vi "addCoolingBars.vi"() -> ()   [LabVIEW 2015]
uses:
  GlobalPath.vi
  GlobalData.vi
  GlobalVi.vi
panel:
  in  "Done?":bool
  in  "ptfe 2":bool caption="Position the 2 cooling bars"
  in  "Save the IDs in the database?":bool
  in  "Fill database with all cooling bar IDs?\nFill database with all 10 frame IDs?\nTo do so go to the database, select the Frame tab, choose the correct frame ID and press \"check_db\"\nThen click on \"Add/Update Entry\"":bool
  in  "COOLING BAR 2":string
  in  "COOLING BAR 1":string
  # "Add cooling bars"
  # "Associate the cooling bars to the panel in the database"
  # "Scan the ID of each of the cooling bars and associate them with the panel"
  # "Cooling bar ID recording"
  # "Fill each box with the correct IDs and press SAVE"
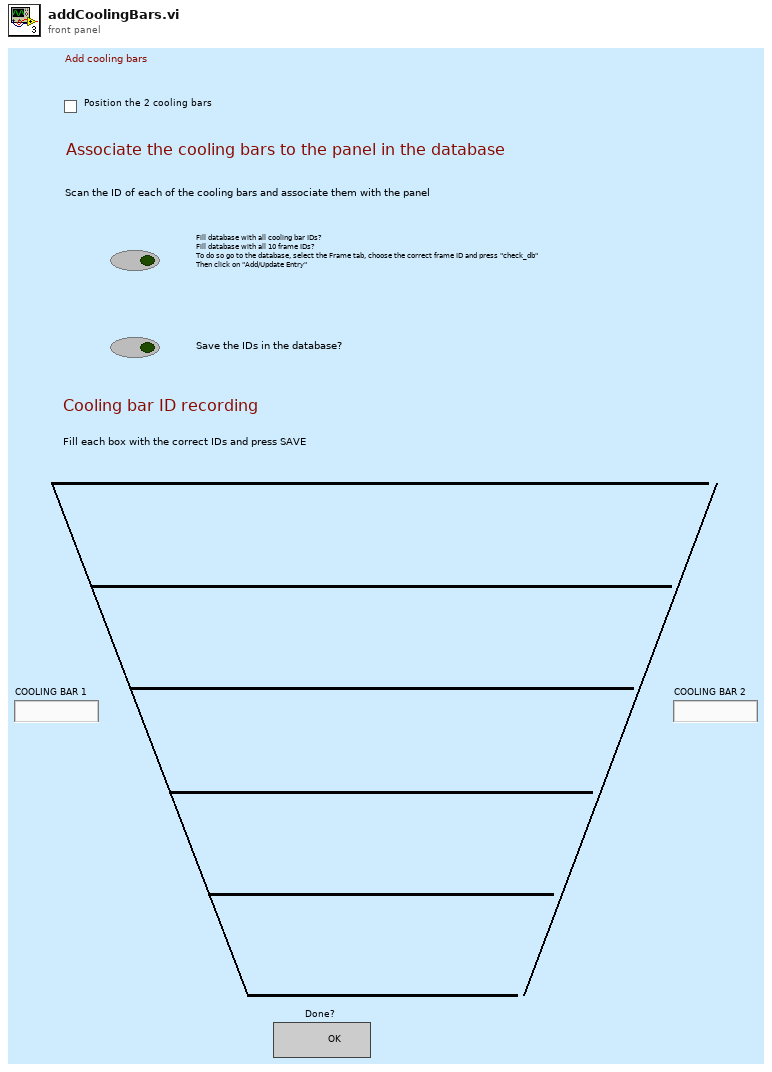
[diagram p1: front panel]
types:
  T1 = enum16{"open", "replace", "create", "open or create", "replace or create", "replace or create with confirmation"}
  T2 = enum32{"Bad", "Idle", "Run top level", "Running"}
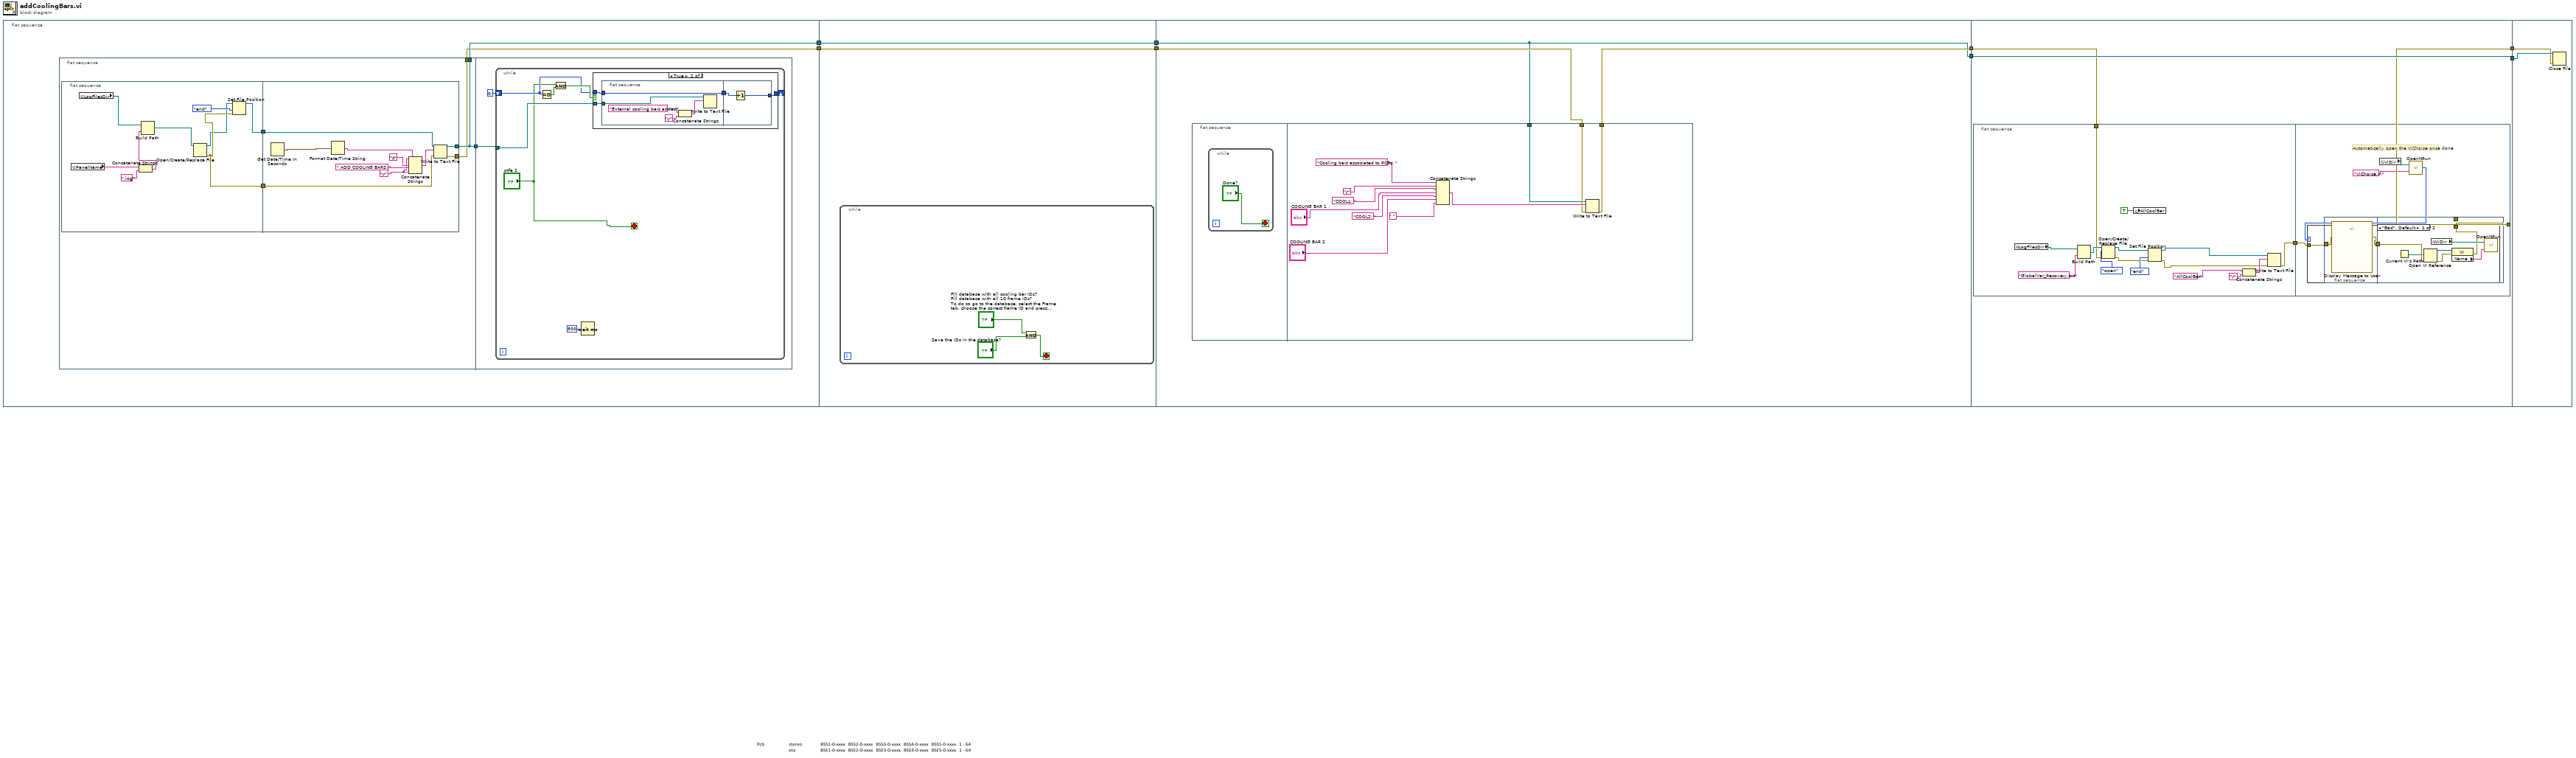
[diagram p0: block diagram]
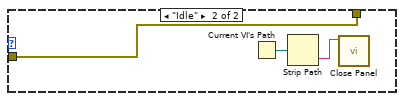
[diagram p3: hidden frame]
diagram:
  n1 = flat-sequence {
    tunnel: [w10] -> w8
    tunnel: [w9] -> w7
    tunnel: w8 -> [w57]
    tunnel: [w57] -> w2
    tunnel: w7 -> [w56]
    tunnel: [w56] -> w1
    tunnel: w2 -> [w61]
    tunnel: [w62] -> w5
    tunnel: w1 -> [w63]
    tunnel: [w61] -> w4
    tunnel: [w78] -> w6
    tunnel: w5 -> [w77]
    tunnel: w4 -> [w79]
    tunnel: [w79] -> w3
    tunnel: w6 -> [w115]
    tunnel: w3 -> [w116]
    frame #0 {
      n2 = flat-sequence {
        tunnel: [w14] -> w11
        tunnel: [w14] -> w10
        tunnel: [w13] -> w9
        tunnel: w11 -> [w36]
        frame #0 {
          n3 = flat-sequence {
            tunnel: [w17] -> w15
            tunnel: [w19] -> w12
            tunnel: w15 -> [w30]
            tunnel: [w29] -> w14
            tunnel: [w28] -> w13
            tunnel: w12 -> [w27]
            frame #0 {
              n4 = global read "GlobalData.vi" "PanelName"() -> (w23:string)
              n5 = global read "GlobalPath.vi" "LogFilesDir"() -> (w16:path)
              n6 = Concatenate Strings(w23, ".log") -> (w22:string)
              n7 = Build Path(base path=w16, name or relative path=w22) -> (appended path=w21:path)
              n8 = Open/Create/Replace File(file path (use dialog)=w21) -> (refnum out=w18:refnum<file>, error out=w19:errorcluster)  [unwired: 5 in, 1 out]
              n9 = Set File Position(refnum=w18, from (0:start)=enum16{"start", "end", "current"}."end", error in=w19) -> (refnum out=w17:refnum<file>)  [unwired: 1 in, 1 out]
            }
            frame #1 {
              w26 = "\r"
              n10 = Get Date/Time In Seconds() -> (seconds since 1Jan1904=w25:timestamp)
              n11 = Format Date/Time String(seconds (now)=w25) -> (date/time string=w32:string)  [unwired: 2 in]
              n12 = Concatenate Strings(w26, w32, "\t", " ADD COOLING BARS: ", w26) -> (w31:string)
              n13 = Write to Text File(file (use dialog)=w30, text=w31, error in=w27) -> (refnum out=w29:refnum<file>, error out=w28:errorcluster)  [unwired: 1 in, 1 out]
            }
          }
        }
        frame #1 {
          n14 = while {
            tunnel: w36 -> [w38]
            shift-right: [w39] -> _
            shift-left: 0 -> [w40]
            stop <- "ptfe 2" stop-if-true
            n15 = Equal To 0?(x=w40) -> (x = 0?=w42:bool)
            n16 = And(x="ptfe 2", y=w42) -> (x .and. y?=w41:bool)
            n17 = Wait (ms)(milliseconds to wait=u32 500) -> ()  [unwired: 1 out]
            n18 = case shown="True" w41 {
              tunnel: w38 -> [_ w48]
              tunnel: w40 -> [w44 w46]
              tunnel: [w44 w45] -> w39
              frame False {
              }
              frame True {
                n19 = flat-sequence {
                  tunnel: w48 -> [w50]
                  tunnel: [w49] -> w47
                  tunnel: w46 -> [w49]
                  tunnel: w47 -> [w55]
                  tunnel: [w54] -> w45
                  frame #0 {
                    n20 = Concatenate Strings("External cooling bars added", "\r") -> (w53:string)
                    n21 = Write to Text File(file (use dialog)=w50, text=w53) -> ()  [unwired: 2 in, 3 out]
                  }
                  frame #1 {
                    n22 = Increment(x=w55) -> (x+1=w54:i32)
                  }
                }
              }
            }
          }
        }
      }
    }
    frame #1 {
      n23 = while {
        stop <- w58 stop-if-true
        n24 = And(x="Fill database with all cooling bar IDs?\nFill database with all 10 frame IDs?\nTo do so go to the database, select the Frame tab, choose the correct frame ID and press \"check_db\"\nThen click on \"Add/Update Entry\"", y="Save the IDs in the database?") -> (x .and. y?=w58:bool)
      }
    }
    frame #2 {
      n25 = flat-sequence {
        tunnel: w63 -> [w72]
        tunnel: w61 -> [w71]
        tunnel: [w70] -> w62
        frame #0 {
          n26 = while {
            stop <- "Done?" stop-if-true
          }
        }
        frame #1 {
          n27 = Concatenate Strings("Cooling bars associated to PCBs: ", "\r", "COOL1: ", "COOLING BAR 1", "COOL2: ", "COOLING BAR 2", " ") -> (w73:string)
          n28 = Write to Text File(file (use dialog)=w71, text=w73, error in=w72) -> (error out=w70:errorcluster)  [unwired: 1 in, 2 out]
        }
      }
    }
    frame #3 {
      n29 = flat-sequence {
        tunnel: w77 -> [w83]
        tunnel: [w82] -> w76
        tunnel: [w96] -> w78
        tunnel: w76 -> [w95]
        frame #0 {
          n30 = global read "GlobalPath.vi" "LogFilesDir"() -> (w80:path)
          n31 = Build Path(base path=w80, name or relative path="GlobalVar_Recovery.txt") -> (appended path=w92:path)
          n32 = Open/Create/Replace File(file path (use dialog)=w92, error in=w83, operation (0:open)=T1."open") -> (refnum out=w88:refnum<file>, error out=w89:errorcluster)  [unwired: 3 in, 1 out]
          n33 = global write "GlobalVi.vi" "AllCoolBar"(TRUE) -> ()
          n34 = Set File Position(refnum=w88, from (0:start)=enum16{"start", "end", "current"}."end", error in=w89) -> (refnum out=w85:refnum<file>, error out=w84:errorcluster)  [unwired: 1 in]
          n35 = Concatenate Strings("AllCoolBar", "\r") -> (w87:string)
          n36 = Write to Text File(file (use dialog)=w85, text=w87, error in=w84) -> (error out=w82:errorcluster)  [unwired: 1 in, 2 out]
        }
        frame #1 {
          # "Automatically open the ViChoise once done"
          n37 = global read "GlobalPath.vi" "ViDir"() -> (w99:path)
          n38 = call "OpenNRun.vi"("VI name"="ViChoice.vi", "ViDirPath"=w99) -> ("Execution:State"=w98:T2)
          n39 = case shown="\"Bad\", Default" w98 {
            tunnel: [w100 w112] -> w96
            tunnel: w95 -> [w101 w112]
            frame "Bad", Default {
              n40 = flat-sequence {
                tunnel: w101 -> [w104]
                tunnel: [w103] -> w102
                tunnel: w102 -> [w108]
                tunnel: [w105] -> w100
                frame #0 {
                  n41 = call "Display Message to User"("error in (no error)"=w104) -> ("error out"=w103:errorcluster)  [unwired: 9 in, 1 out]
                }
                frame #1 {
                  n42 = Current VI's Path() -> (path=w106:path)
                  n43 = Open VI Reference(vi path=w106, error in (no error)=w108) -> (vi reference=w111:refnum<vi>, error out=w110:errorcluster)  [unwired: 4 in]
                  n44 = global read "GlobalPath.vi" "ViDir"() -> (w107:path)
                  n45 = property class="VI"(reference=w111, error in=w110) -> (error out=w105:errorcluster, "Name"=w109:string)  [unwired: 1 out]
                  n46 = call "OpenNRun.vi"("VI name"=w109, "ViDirPath"=w107) -> ()  [unwired: 1 out]
                }
              }
            }
            frame "Idle" {
              n47 = Current VI's Path() -> (path=w113:path)
              n48 = Strip Path(path=w113) -> (name=w114:string)  [unwired: 1 out]
              n49 = call <vilib>:"Close Panel.vi"("VI name"=w114) -> ()  [unwired: 10 in, 1 out]
            }
          }
        }
      }
    }
    frame #4 {
      n50 = Close File(refnum=w116, error in=w115) -> ()  [unwired: 2 out]
    }
  }
